vi "Close.vi"(8 "error in (no error)":errorcluster) -> (0 "error out":errorcluster)   [LabVIEW 2020, in "My Cloneable Module.lvlib" / "VI Reference Management.lvlib"]
doc: "Close the master reference of the cloneable Main VI.\n_____\nBased on DQMH Project Template 6.0.0.91."
uses:
  VI Reference Management.lvlib
  Action--enum.ctl
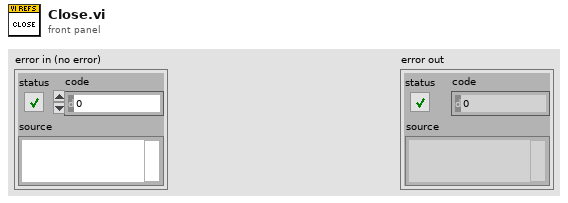
[diagram p1: front panel]
types:
  T1 = typedef "My Cloneable Module.lvlib/VI Reference Management.lvlib/Action--enum.ctl" = enum16{"Get", "Create", "Close"}
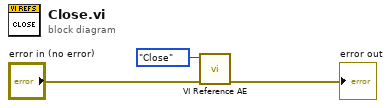
[diagram p0: block diagram]
diagram:
  n1 = call "VI Reference AE.vi"("error in (no error)"="error in (no error)", "Action"=Action--enum."Close") -> ("error out"=→"error out":errorcluster)  [unwired: 7 in, 1 out]
